vi "BPS Driver.vi"(9 "Supply Voltage":fxp<+/-,24,5>, 11 "Signal In":fxp<+/-,26,5>) -> (2 "Brake Pressure (psi)":fxp<+,26,13>, 3 "Sensor OK?":bool)   [LabVIEW 2015]
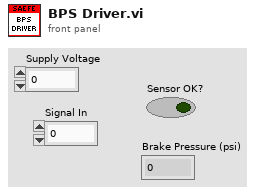
[diagram p1: front panel]
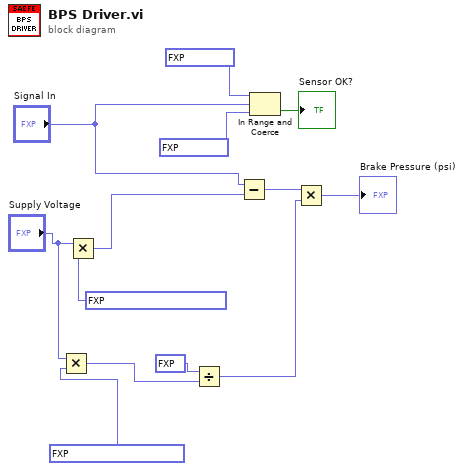
[diagram p0: block diagram]
diagram:
  n1 = Multiply(x="Supply Voltage", y=fxp<+,26,5> 0.8000001907348633) -> (x*y=w3:fxp<+,26,4>)
  n2 = Multiply(x="Supply Voltage", y=fxp<+/-,26,5> 0.09999990463256836) -> (x*y=w6:fxp<+,16,2>)
  n3 = Divide(x=fxp<+,26,26> 5000.0, y=w3) -> (x/y=w1:fxp<+,26,10>)
  n4 = Subtract(x="Signal In", y=w6) -> (x-y=w12:fxp<+,27,5>)
  n5 = In Range and Coerce(upper limit=fxp<+/-,14,5> 4.599609375, x="Signal In", lower limit=fxp<+/-,14,5> 0.400390625) -> (In Range?=→"Sensor OK?":bool)  [unwired: 1 out]
  n6 = Multiply(x=w12, y=w1) -> (x*y=→"Brake Pressure (psi)":fxp<+,26,13>)
